vi "FXP Write base.vi"(8 "error in (no error)":errorcluster, 9 "data in":dbl, 10 "integersize":i32, 11 "shared variable refnum in":refnum<k21>) -> (0 "error out":errorcluster, 1 "data out":dbl, 3 "shared variable refnum out":refnum<k21>)   [LabVIEW 2011]
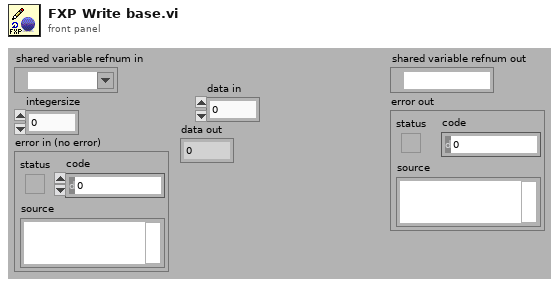
[diagram p1: front panel]
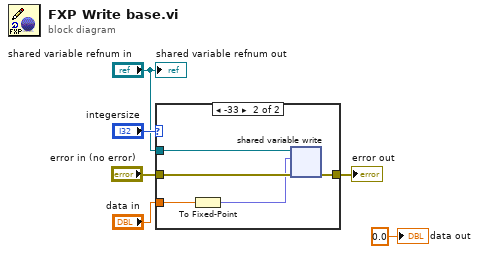
[diagram p0: block diagram]
diagram:
  n1 = case shown="-33" "integersize" {
    tunnel: "error in (no error)" -> [w7 w12]
    tunnel: [w7 w11] -> w4
    tunnel: "shared variable refnum in" -> [_ w10]
    tunnel: "data in" -> [_ w8]
    frame 2048, Default {
    }
    frame -33 {
      n2 = To Fixed-Point(number=w8) -> (fixed-point=w9:fxp<+/-,32,16>)  [unwired: 1 in]
      n3 = shared-variable-write ("Scanned Variable Write")(w10, w12, w9) -> (w11:errorcluster)  [unwired: 1 out]
    }
  }
  "error out" <- w4
  "shared variable refnum out" <- "shared variable refnum in"
  "data out" <- 0.0 ("data out")
